vi "Constructor.vi"(8 "error in (no error)":errorcluster, 11 "Eurotherm 3200 PID Controller in":refnum<class "Eurotherm 3200 PID Controller.lvclass">) -> (0 "error out":errorcluster, 3 "Eurotherm 3200 PID Controller out":refnum<class "Eurotherm 3200 PID Controller.lvclass">)   [LabVIEW 2011, in "Eurotherm 3200 PID Controller.lvclass"]
uses:
  Eurotherm 3200 PID Controller.lvclass
  Eurotherm 3200 PID Controller.lvclass/Eurotherm 3200 PID Controller.ctl
  <instrlib>/Eurotherm 32xx Series/Eurotherm 32xx Series.lvlib
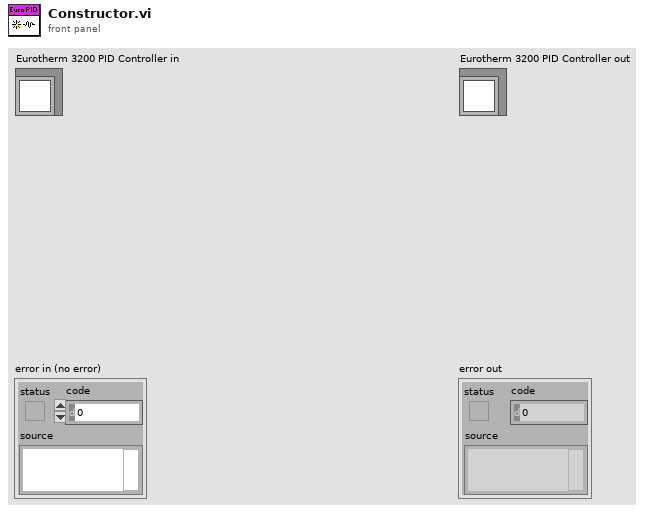
[diagram p1: front panel]
types:
  T1 = cluster{"Baud Rate":u32, "Parity":u16, "Break Length":u16}
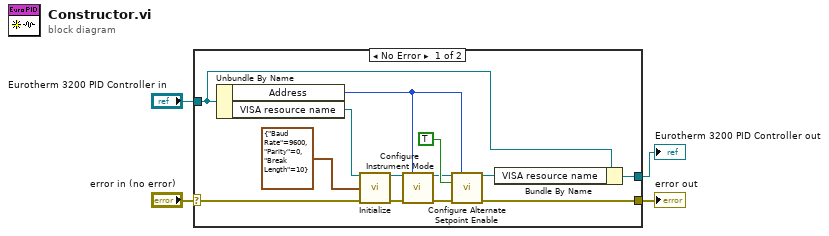
[diagram p0: block diagram]
diagram:
  n1 = case shown="No Error" "error in (no error)" {
    selector: "error in (no error)" -> [w7 w19]
    tunnel: [w6 w19] -> w3
    tunnel: [w5 w18] -> w1
    tunnel: "Eurotherm 3200 PID Controller in" -> [w9 w18]
    frame No Error {
      n2 = Unbundle By Name(w9) -> ("Address"=w10:u8, "VISA resource name"=w11:refnum<visa-resource-name>)
      n3 = call <instrlib>:"Initialize.vi"("VISA resource name"=w11, "Serial Configuration"=T1 {"Baud Rate"=9600, "Parity"=0, "Break Length"=10} ("Serial Config"), "error in (no error)"=w7) -> ("VISA resource name out"=w13:refnum<visa-resource-name>, "error out"=w14:errorcluster)  [unwired: 11 in]
      n4 = call <instrlib>:"Configure Instrument Mode.vi"("VISA resource name"=w13, "Unit Address (1)"=w10, "error in (no error)"=w14) -> ("VISA resource name out"=w15:refnum<visa-resource-name>, "error out"=w16:errorcluster)  [unwired: 11 in]
      n5 = call <instrlib>:"Configure Alternate Setpoint Enable.vi"("VISA resource name"=w15, "Unit Address (1)"=w10, "Enable Alternate Setpoint (False: Disable)"=TRUE, "error in (no error)"=w16) -> ("VISA resource name out"=w8:refnum<visa-resource-name>, "error out"=w6:errorcluster)  [unwired: 10 in]
      n6 = Bundle By Name(cluster=w9, "VISA resource name"=w8) -> (w5:refnum<class "Eurotherm 3200 PID Controller.lvclass">)
    }
    frame Error {
    }
  }
  "error out" <- w3
  "Eurotherm 3200 PID Controller out" <- w1
